vi "Structures.vi"(7 "PythonConverter_BD in":refnum<class "PyConvBD.lvclass">, 8 "error in":errorcluster, 11 "Diagram in":refnum<class "Diagram.lvclass">) -> (0 "error out":errorcluster, 3 "Diagram out":refnum<class "Diagram.lvclass">, 4 "structures":string, 5 "PythonConverter_BD out":refnum<class "PyConvBD.lvclass">)   [LabVIEW 2014, in "Raspberry Pi Compatible Compiler for LabVIEW.lvlib" / "Diagram.lvclass"]
uses:
  Diagram.lvclass
  Python/PythonConverter_BD/PyConvBD.lvclass
  Diagram.lvclass/Diagram.ctl
  <vilib>/Utility/error.llb/whitespace.ctl
  Structure/Structure.lvclass
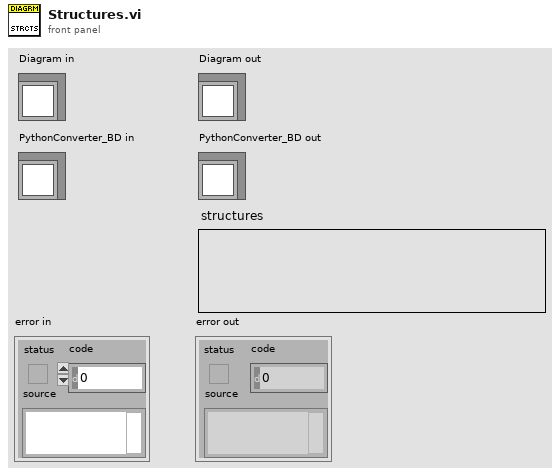
[diagram p1: front panel]
types:
  T1 = typedef "whitespace.ctl" = u16
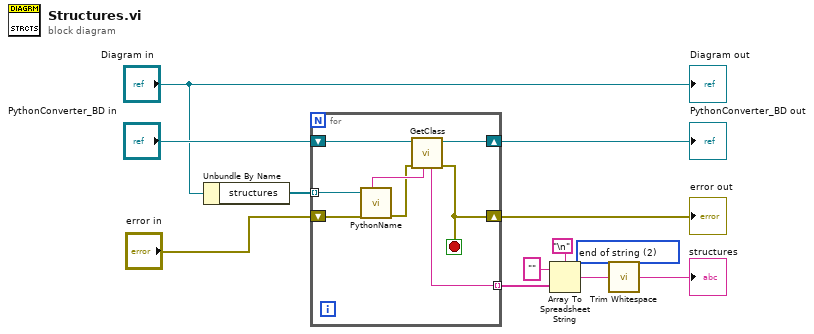
[diagram p0: block diagram]
diagram:
  w3 = T1 2 items=["both", "start of string", "end of string"] ("location (both)")
  n1 = Unbundle By Name("Diagram in") -> ("structures"=w12:refnum<class "Structure.lvclass">[])
  n2 = for {
    tunnel: w12 -> [w17] mode=indexing
    shift-right: [w20] -> w9
    shift-left: "PythonConverter_BD in" -> [w19]
    shift-right: [w14] -> w7
    shift-left: "error in" -> [w18]
    tunnel: [w13] -> w2 mode=indexing
    stop <- w14 stop-if-true
    n3 = call-dynamic "PythonName.vi"("error in"=w18, "Node in"=w17) -> ("error out"=w15:errorcluster, "UID"=w16:string)  [unwired: 6 in, 2 out]
    n4 = call "GetClass.vi"("name"=w16, "error in"=w15, "PythonConverter_BD in"=w19) -> ("error out"=w14:errorcluster, "PythonConverter_BD out"=w20:refnum<class "PyConvBD.lvclass">, "class"=w13:string)  [unwired: 4 in]
  }
  "error out" <- w7
  "PythonConverter_BD out" <- w9
  n5 = Array To Spreadsheet String(delimiter (Tab)="\n", array=w2, 3:"" ("format string")) -> (spreadsheet string=w4:string)
  n6 = call <vilib>:"Trim Whitespace.vi"("string"=w4, "location (both)"=w3) -> ("trimmed string"=→"structures":string)
  "Diagram out" <- "Diagram in"
